vi "Test Has Events.vi"(8 "error in (no error)":errorcluster) -> (0 "error out":errorcluster)   [LabVIEW 2020, in "TEST JKI State Machine API.lvlib"]
uses:
  TEST JKI State Machine API.lvlib
  source/JKI SM/JKI SM.lvclass
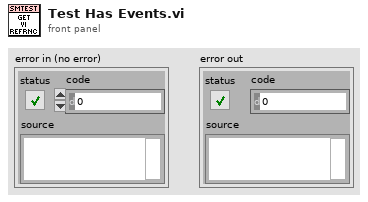
[diagram p1: front panel]
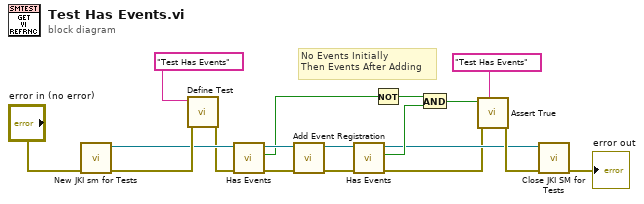
[diagram p0: block diagram]
diagram:
  # "No Events Initially\nThen Events After Adding"
  n1 = call "New JKI sm for Tests.vi"("error in (no error)"="error in (no error)") -> ("error out"=w13:errorcluster, "JKI SM out"=w12:refnum<class "JKI SM.lvclass">)  [unwired: 9 in]
  n2 = call <vilib>:"Define Test.vi"("error in (no error)"=w13, "Label (VI Title)"="Test Has Events") -> ("error out"=w11:errorcluster)  [unwired: 8 in, 1 out]
  n3 = call "Has Events.vi"("error in (no error)"=w11, "JKI SM in"=w12) -> ("error out"=w10:errorcluster, "Registered for Events?"=w5:bool, "JKI SM out"=w9:refnum<class "JKI SM.lvclass">)  [unwired: 7 in]
  n4 = call-dynamic "Add Event Registration.vi"("error in (no error)"=w10, "JKI SM in"=w9) -> ("error out"=w8:errorcluster, "JKI SM out"=w7:refnum<class "JKI SM.lvclass">)  [unwired: 8 in]
  n5 = call "Has Events.vi"("error in (no error)"=w8, "JKI SM in"=w7) -> ("error out"=w2:errorcluster, "Registered for Events?"=w4:bool, "JKI SM out"=w3:refnum<class "JKI SM.lvclass">)  [unwired: 7 in]
  n6 = Not(x=w5) -> (.not. x?=w6:bool)
  n7 = And(x=w6, y=w4) -> (x .and. y?=w1:bool)
  n8 = call <vilib>:"Assert True.vi"("Label"="Test Has Events", "error in (no error)"=w2, "True?"=w1) -> ("error out"=w16:errorcluster)  [unwired: 7 in, 1 out]
  n9 = call "Close JKI SM for Tests.vi"("error in (no error)"=w16, "JKI SM in"=w3) -> ("error out"=→"error out":errorcluster)  [unwired: 9 in]
